vi "Simple Example.vi"() -> ()   [LabVIEW 2023]
panel:
  out "Error Out":errorcluster
  in  "stop":bool
  out "Total Power":dbl
  out "DOP":dbl
  out "s1":dbl
  out "s2":dbl
  out "s3":dbl
  out "Ellipticity deg":dbl caption="Ellipticity rad"
  out "Azimuth deg":dbl caption="Azimuth rad"
  in  "Wavelength":dbl=6.36e-07
  in  "Basic Scan Rate":dbl=66.0
  in  "Autorange":bool=TRUE caption="Autorange (On)"
  in  "Operation Mode":i32(ring)=5 caption="Mode (Double Waveplate Rotation - 2048 Point FFT)" items=["Idle", "Half Waveplate Rotation - 512 Point FFT", "Half Waveplate Rotation - 1024 Point FFT", "Half Waveplate Rotation - 2048 Point FFT", "Full Waveplate Rotation - 512 Point FFT", "Full Waveplate Rotation - 1024 Point FFT", "Full Waveplate Rotation - 2048 Point FFT", "Double Waveplate Rotation - 512 Point FFT", "Double Waveplate Rotation - 1024 Point FFT", "Double Waveplate Rotation - 2048 Point FFT"]
  out "S/N":string
  out "Device Name":string
  in  "Error In":errorcluster
  # "Device"
  # "Settings"
  # "Measurement Results"
  # "Status"
  # "Stop Program"
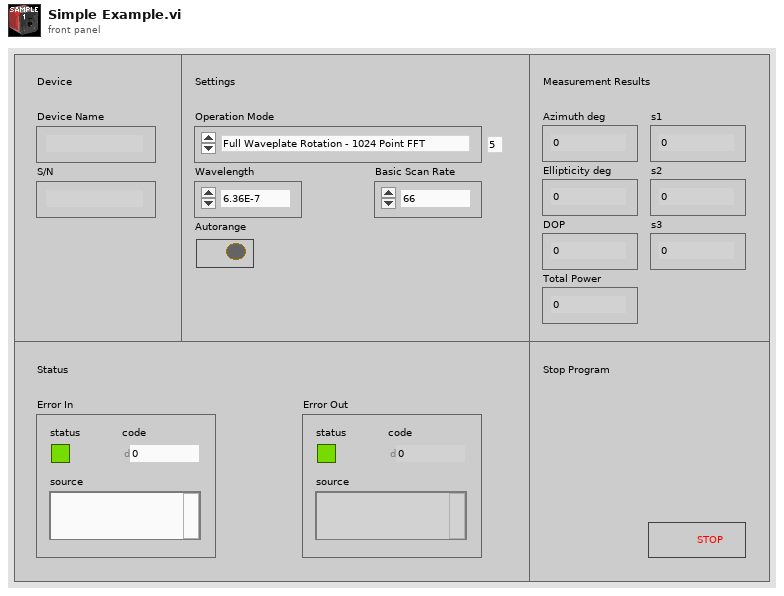
[diagram p1: front panel]
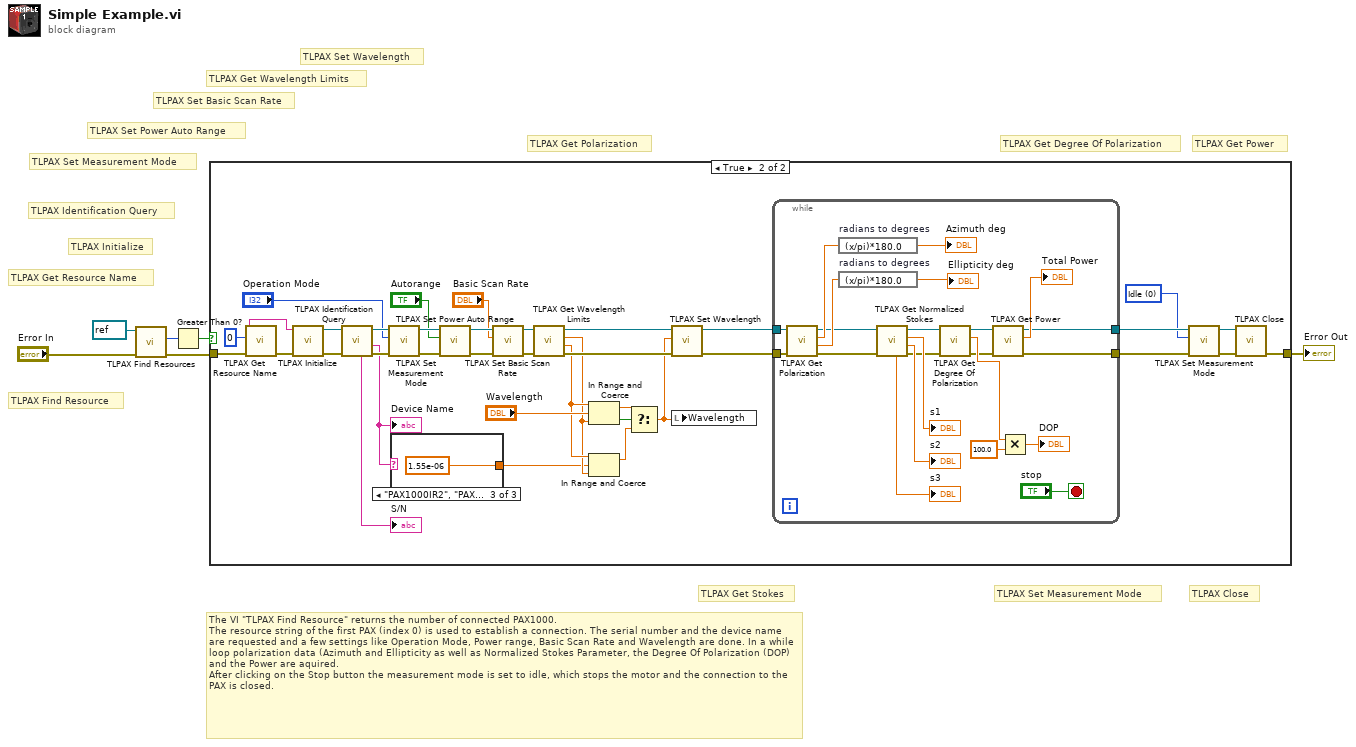
[diagram p0: block diagram]
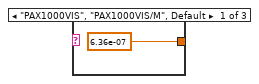
[diagram p3: hidden frame]
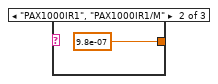
[diagram p4: hidden frame]
diagram:
  # "The VI \"TLPAX Find Resource\" returns the number of connected PAX1000.\nThe resource string of the first PAX (index 0) is used to establish a connection. The serial number and the device name are requested and a few settings like Operation Mode, Power range, Basic Scan Rate and Wavelength are done. In a while loop polarization data (Azimuth and Ellipticity as well as Normalized Stokes Parameter, the Degree Of Polarization (DOP) and the Power are aquired.\nAfter clicking on the Stop button the measurement mode is set to idle, which stops the motor and the connection to the PAX is closed."
  # "TLPAX Set Measurement Mode"
  # "TLPAX Close"
  # "TLPAX Set Measurement Mode"
  # "TLPAX Get Power"
  # "TLPAX Get Degree Of Polarization"
  # "TLPAX Get Stokes"
  # "TLPAX Get Polarization"
  # "TLPAX Set Wavelength"
  # "TLPAX Get Wavelength Limits"
  # "TLPAX Set Basic Scan Rate"
  # "TLPAX Set Power Auto Range"
  # "TLPAX Identification Query"
  # "TLPAX Initialize"
  # "TLPAX Get Resource Name"
  # "TLPAX Find Resource"
  n1 = call <instrlib>:"TLPAX Find Resources.vi"("error in (no error)"="Error In", "instrument handle"=refnum<visa-resource-name> refnum) -> ("error out"=w2:errorcluster, "Device Count"=w5:u32)  [unwired: 7 in, 1 out]
  n2 = Greater Than 0?(x=w5) -> (x > 0?=w4:bool)
  n3 = case shown="True" w4 {
    tunnel: w2 -> [w7 w43]
    tunnel: [w7 w22] -> w1
    frame False {
    }
    frame True {
      w28 = 0 items=["Idle", "Half Waveplate Rotation - 512 Point FFT", "Half Waveplate Rotation - 1024 Point FFT", "Half Waveplate Rotation - 2048 Point FFT", "Full Waveplate Rotation - 512 Point FFT", "Full Waveplate Rotation - 1024 Point FFT", "Full Waveplate Rotation - 2048 Point FFT", "Double Waveplate Rotation - 512 Point FFT", "Double Waveplate Rotation - 1024 Point FFT", "Double Waveplate Rotation - 2048 Point FFT"] ("Mode (Double Waveplate Rotation - 2048 Point FFT)")
      n4 = call <instrlib>:"TLPAX Get Resource Name.vi"("error in (no error)"=w43, "Index (0)"=u32 0) -> ("error out"=w42:errorcluster, "Resource Name"=w41:string)  [unwired: 7 in, 1 out]
      n5 = call <instrlib>:"TLPAX Initialize.vi"("error in (no error)"=w42, "resource name"=w41) -> ("error out"=w40:errorcluster, "instrument handle out"=w39:refnum<visa-resource-name>)  [unwired: 8 in]
      n6 = call <instrlib>:"TLPAX Identification Query.vi"("error in (no error)"=w40, "instrument handle"=w39) -> ("error out"=w37:errorcluster, "Device Name"=w16:string, "instrument handle out"=w36:refnum<visa-resource-name>, "Serial Number"=→"S/N":string)  [unwired: 4 in, 2 out]
      "Device Name" <- w16
      n7 = call <instrlib>:"TLPAX Set Measurement Mode.vi"("error in (no error)"=w37, "Mode (Double Waveplate Rotation - 2048 Point FFT)"="Operation Mode", "instrument handle"=w36) -> ("error out"=w34:errorcluster, "instrument handle out"=w33:refnum<visa-resource-name>)  [unwired: 7 in]
      n8 = case shown="\"PAX1000IR2\", \"PAX1000IR2/M\"" w16 {
        tunnel: [6.36e-07 ("Wavelength") 9.8e-07 ("Wavelength") 1.55e-06 ("Wavelength")] -> w12
        frame "PAX1000VIS", "PAX1000VIS/M", Default {
        }
        frame "PAX1000IR1", "PAX1000IR1/M" {
        }
        frame "PAX1000IR2", "PAX1000IR2/M" {
        }
      }
      n9 = call <instrlib>:"TLPAX Set Power Auto Range.vi"("error in (no error)"=w34, "Autorange (On)"="Autorange", "instrument handle"=w33) -> ("error out"=w27:errorcluster, "instrument handle out"=w26:refnum<visa-resource-name>)  [unwired: 7 in]
      n10 = call <instrlib>:"TLPAX Set Basic Scan Rate.vi"("error in (no error)"=w27, "Basic Scan Rate"="Basic Scan Rate", "instrument handle"=w26) -> ("error out"=w19:errorcluster, "instrument handle out"=w20:refnum<visa-resource-name>)  [unwired: 7 in]
      n11 = call <instrlib>:"TLPAX Get Wavelength Limits.vi"("error in (no error)"=w19, "instrument handle"=w20) -> ("error out"=w18:errorcluster, "Maximum"=w14:dbl, "Minimum"=w13:dbl, "instrument handle out"=w17:refnum<visa-resource-name>)  [unwired: 6 in]
      n12 = In Range and Coerce(upper limit=w14, x="Wavelength", lower limit=w13) -> (coerced(x)=w10:dbl, In Range?=w11:bool)
      n13 = In Range and Coerce(upper limit=w14, x=w12, lower limit=w13) -> (coerced(x)=w9:dbl)  [unwired: 1 out]
      n14 = Select(t=w10, s=w11, f=w9) -> (s? t:f=w8:dbl)
      n15 = call <instrlib>:"TLPAX Set Wavelength.vi"("error in (no error)"=w18, "Wavelength"=w8, "instrument handle"=w17) -> ("error out"=w21:errorcluster, "instrument handle out"=w31:refnum<visa-resource-name>)  [unwired: 7 in]
      n16 = local write "Wavelength"(w8) -> ()
      n17 = while {
        tunnel: w31 -> [w57]
        tunnel: w21 -> [w56]
        tunnel: [w55] -> w30
        tunnel: [w50] -> w29
        stop <- "stop" stop-if-true
        n18 = call <instrlib>:"TLPAX Get Polarization.vi"("error in (no error)"=w56, "instrument handle"=w57) -> ("error out"=w48:errorcluster, "Ellipticity rad"=w66:dbl, "Azimuth rad"=w67:dbl, "instrument handle out"=w49:refnum<visa-resource-name>)  [unwired: 6 in]
        n19 = expression code="(x/pi)*180.0" "radians to degrees"(w67) -> (→"Azimuth deg":dbl)
        n20 = expression code="(x/pi)*180.0" "radians to degrees"(w66) -> (→"Ellipticity deg":dbl)
        n21 = call <instrlib>:"TLPAX Get Normalized Stokes.vi"("error in (no error)"=w48, "instrument handle"=w49) -> ("error out"=w54:errorcluster, "s2"=→"s2":dbl, "s1"=→"s1":dbl, "instrument handle out"=w53:refnum<visa-resource-name>, "s3"=→"s3":dbl)  [unwired: 5 in]
        n22 = call <instrlib>:"TLPAX Get Degree Of Polarization.vi"("error in (no error)"=w54, "instrument handle"=w53) -> ("error out"=w52:errorcluster, "DOP"=w61:dbl, "instrument handle out"=w51:refnum<visa-resource-name>)  [unwired: 5 in, 2 out]
        n23 = call <instrlib>:"TLPAX Get Power.vi"("error in (no error)"=w52, "instrument handle"=w51) -> ("error out"=w50:errorcluster, "Total Power"=→"Total Power":dbl, "instrument handle out"=w55:refnum<visa-resource-name>)  [unwired: 5 in, 2 out]
        n24 = Multiply(x=w61, y=100.0) -> (x*y=→"DOP":dbl)
      }
      n25 = call <instrlib>:"TLPAX Set Measurement Mode.vi"("error in (no error)"=w29, "Mode (Double Waveplate Rotation - 2048 Point FFT)"=w28, "instrument handle"=w30) -> ("error out"=w23:errorcluster, "instrument handle out"=w24:refnum<visa-resource-name>)  [unwired: 7 in]
      n26 = call <instrlib>:"TLPAX Close.vi"("error in (no error)"=w23, "instrument handle"=w24) -> ("error out"=w22:errorcluster)  [unwired: 9 in]
    }
  }
  "Error Out" <- w1
